vi "Read NI-Scope Lock-in Configuration.vi"(8 "error in (no error)":errorcluster, 11 "NI-Scope Lock-in Driver in":refnum<class "NI-Scope Lock-in Driver.lvclass">) -> (0 "error out":errorcluster, 2 "Configuration":T1={"Points per sine wave"=0, "Rate"=1000000.0, "Re-name channels"=[], "Active channels"="0:1", "Ranges"=[10.0], "Sync on trigger"=FALSE, "R-Q"=FALSE} {"Ranges" format="%#_6pV"; "Rate" format="%#_8pHz"}, 3 "NI-Scope Lock-in Driver out":refnum<class "NI-Scope Lock-in Driver.lvclass">)   [LabVIEW 2016, in "NI-Scope Lock-in Driver.lvclass"]
uses:
  NI-Scope Lock-in Driver.lvclass
  C:/github/NHMFL_Core/Libraries/Instruments/Instrument Driver/Instrument Driver.lvclass
  NI-Scope Lock-in Configuration.ctl
  Instruments/Instrument Driver/Read User configuration.vi
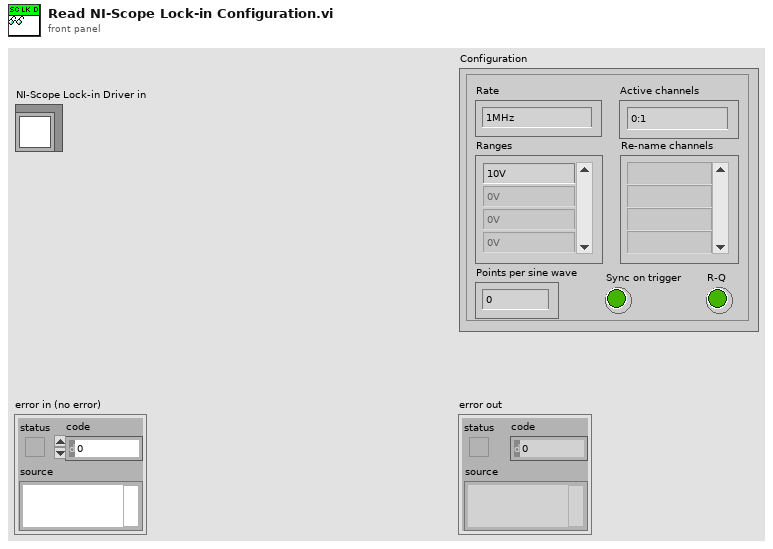
[diagram p1: front panel]
types:
  T1 = typedef "NI-Scope Lock-in Configuration.ctl" = cluster{"Points per sine wave":i32, "Rate":dbl, "Re-name channels":string[], "Active channels":string, "Ranges":dbl[], "Sync on trigger":bool, "R-Q":bool}
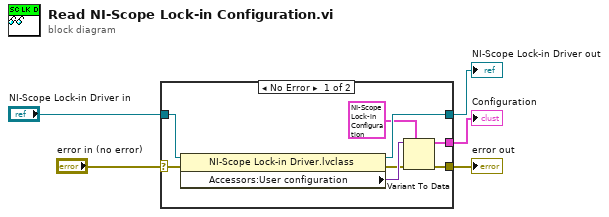
[diagram p0: block diagram]
diagram:
  n1 = case shown="No Error" "error in (no error)" {
    selector: "error in (no error)" -> [w13 w14]
    tunnel: [w6 w14] -> w4
    tunnel: [w11 w15] -> w2
    tunnel: "NI-Scope Lock-in Driver in" -> [w12 w15]
    tunnel: [w8 _] -> w1
    frame No Error {
      n2 = property class="NI-Scope Lock-in Driver.lvclass"(reference=w12, error in=w13) -> (reference out=w11:refnum<class "NI-Scope Lock-in Driver.lvclass">, error out=w7:errorcluster, "Accessors:User configuration"=w10:variant)
      n3 = Variant To Data(error in=w7, type=T1 {"Points per sine wave"=0, "Rate"=1000000.0, "Re-name channels"=[], "Active channels"="0:1", "Ranges"=[10.0], "Sync on trigger"=FALSE, "R-Q"=FALSE} ("Configuration"), Variant=w10) -> (data=w8:T1, error out=w6:errorcluster)
    }
    frame Error {
    }
  }
  "error out" <- w4
  "NI-Scope Lock-in Driver out" <- w2
  "Configuration" <- w1
